vi "4 way traffic light system.vi"() -> ()   [LabVIEW 2021]
panel:
  in  "?":bool
  out "GREEN-S":bool
  out "YELLOW-S":bool
  out "RED-S":bool
  out "GREEN-N":bool
  out "YELLOW-N":bool
  out "RED-N":bool
  out "GREEN-E":bool
  out "YELLOW-E":bool
  out "RED-E":bool
  out "GREEN-W":bool
  out "YELLOW-W":bool
  out "RED-W":bool
  # "-----------------------------------------------------------------------------"
  # "----------------------------------------------------------------"
  # "----------------------------------------------------------------"
  # "------------------------------------------------------------------------"
  # "-------------------------------------------------------------"
  # "-----------------------------------------------------------------------"
  # "---------------------------------------------------------------"
  # "---------------------------------------------------------------"
  # "-------------------------------------------------------------------------"
  # "--------------------------------------------"
  # "-----------------------------------------------"
  # "---------------------------------------------------"
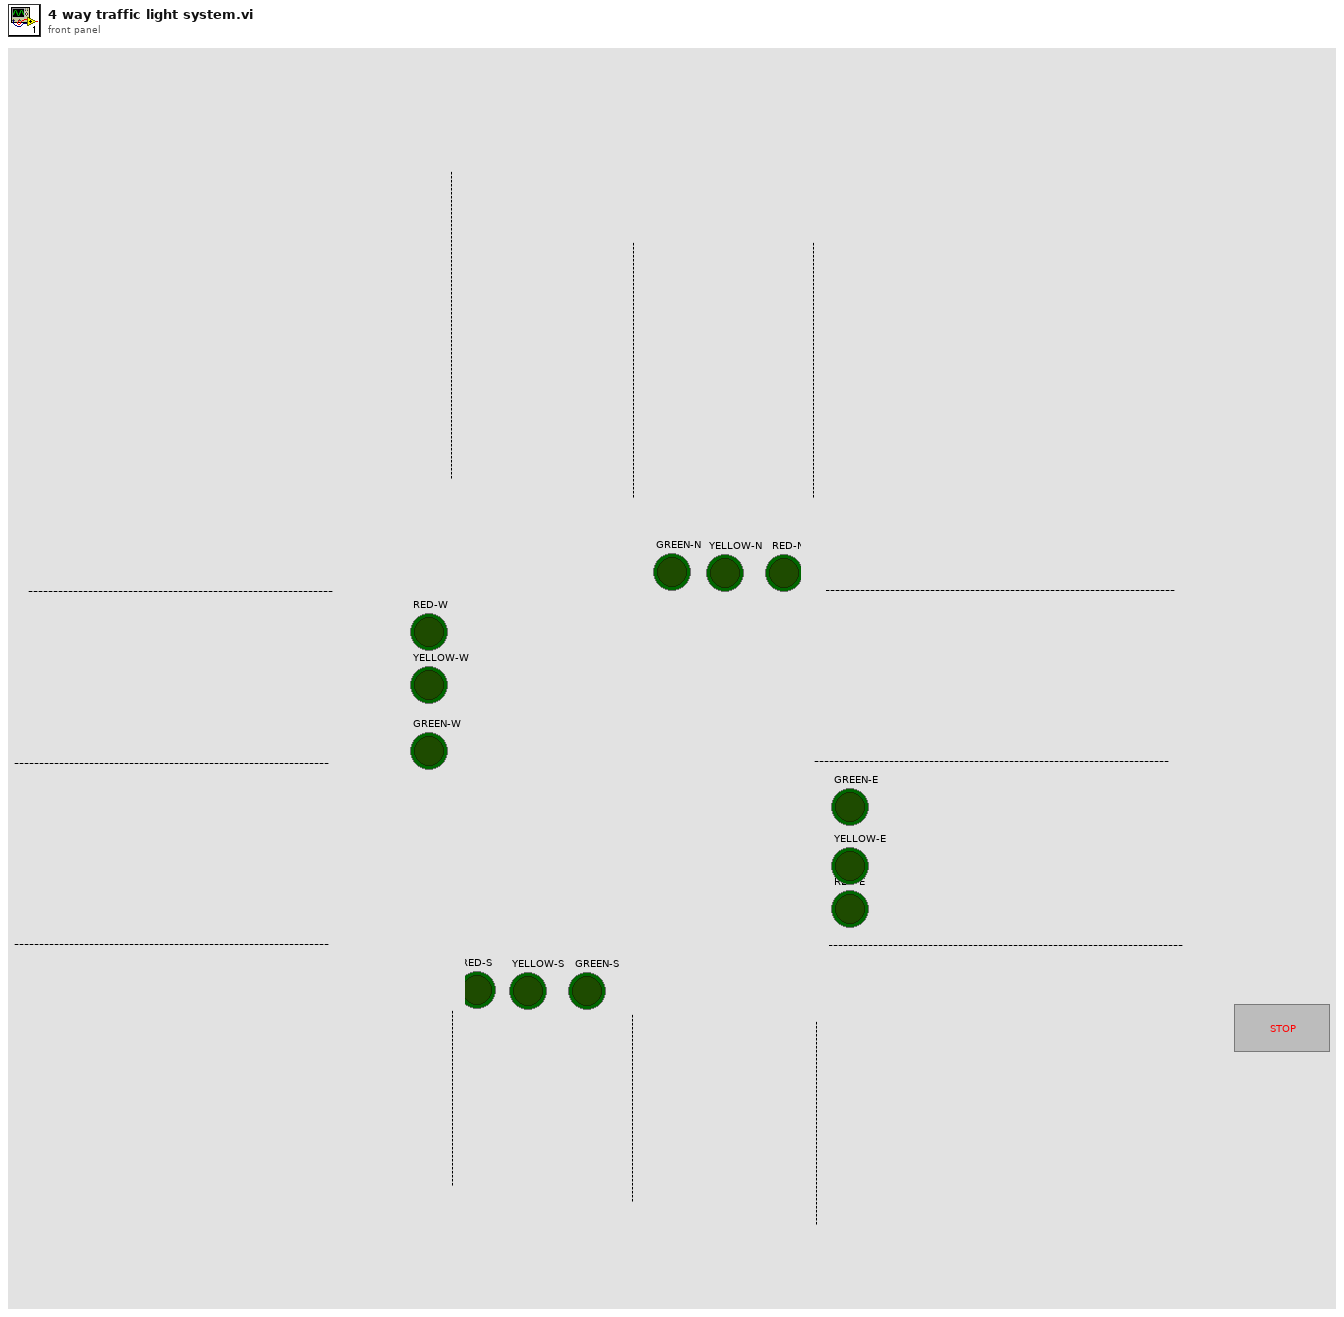
[diagram p1: front panel]
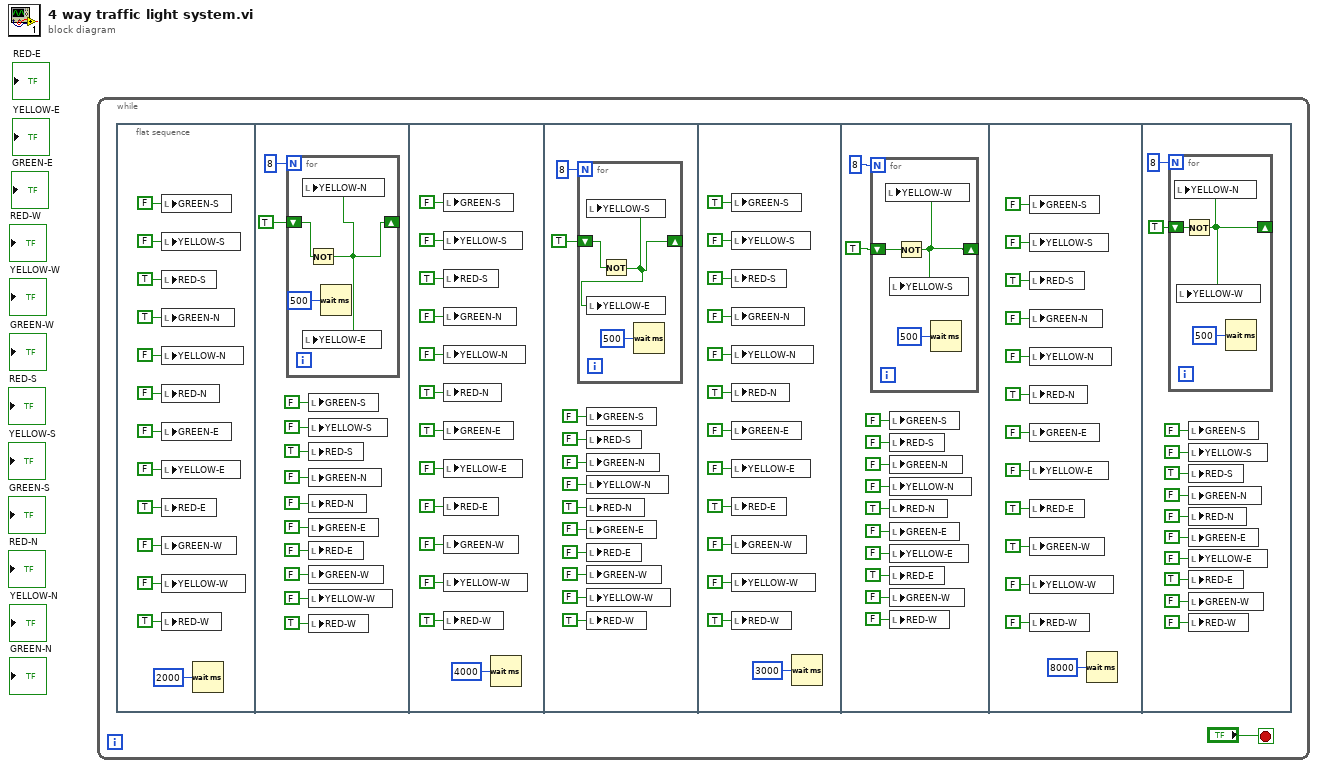
[diagram p0: block diagram]
diagram:
  n1 = while {
    stop <- "?" stop-if-true
    n2 = flat-sequence {
      frame #0 {
        n3 = local write "GREEN-S"(FALSE ("GREEN-S")) -> ()
        n4 = local write "YELLOW-S"(FALSE ("YELLOW-S")) -> ()
        n5 = local write "RED-S"(TRUE ("RED-S")) -> ()
        n6 = local write "GREEN-N"(TRUE ("GREEN-N")) -> ()
        n7 = local write "YELLOW-N"(FALSE ("YELLOW-N")) -> ()
        n8 = local write "RED-N"(FALSE ("RED-N")) -> ()
        n9 = local write "GREEN-E"(FALSE ("GREEN-E")) -> ()
        n10 = local write "YELLOW-E"(FALSE ("YELLOW-E")) -> ()
        n11 = local write "RED-E"(TRUE ("RED-E")) -> ()
        n12 = local write "GREEN-W"(FALSE ("GREEN-W")) -> ()
        n13 = local write "YELLOW-W"(FALSE ("YELLOW-W")) -> ()
        n14 = local write "RED-W"(TRUE ("RED-W")) -> ()
        n15 = Wait (ms)(milliseconds to wait=u32 2000) -> ()  [unwired: 1 out]
      }
      frame #1 {
        n16 = for {
          N: 8 -> [_]
          shift-right: [w27] -> _
          shift-left: TRUE -> [w28]
          n17 = Not(x=w28) -> (.not. x?=w27:bool)
          n18 = local write "YELLOW-N"(w27) -> ()
          n19 = local write "YELLOW-E"(w27) -> ()
          n20 = Wait (ms)(milliseconds to wait=u32 500) -> ()  [unwired: 1 out]
        }
        n21 = local write "GREEN-S"(FALSE ("GREEN-S")) -> ()
        n22 = local write "YELLOW-S"(FALSE ("YELLOW-S")) -> ()
        n23 = local write "RED-S"(TRUE ("RED-S")) -> ()
        n24 = local write "GREEN-N"(FALSE ("GREEN-N")) -> ()
        n25 = local write "RED-N"(FALSE ("RED-N")) -> ()
        n26 = local write "GREEN-E"(FALSE ("GREEN-E")) -> ()
        n27 = local write "RED-E"(FALSE ("RED-E")) -> ()
        n28 = local write "GREEN-W"(FALSE ("GREEN-W")) -> ()
        n29 = local write "YELLOW-W"(FALSE ("YELLOW-W")) -> ()
        n30 = local write "RED-W"(TRUE ("RED-W")) -> ()
      }
      frame #2 {
        n31 = local write "GREEN-S"(FALSE ("GREEN-S")) -> ()
        n32 = local write "YELLOW-S"(FALSE ("YELLOW-S")) -> ()
        n33 = local write "RED-S"(TRUE ("RED-S")) -> ()
        n34 = local write "GREEN-N"(FALSE ("GREEN-N")) -> ()
        n35 = local write "YELLOW-N"(FALSE ("YELLOW-N")) -> ()
        n36 = local write "RED-N"(TRUE ("RED-N")) -> ()
        n37 = local write "GREEN-E"(TRUE ("GREEN-E")) -> ()
        n38 = local write "YELLOW-E"(FALSE ("YELLOW-E")) -> ()
        n39 = local write "RED-E"(FALSE ("RED-E")) -> ()
        n40 = local write "GREEN-W"(FALSE ("GREEN-W")) -> ()
        n41 = local write "YELLOW-W"(FALSE ("YELLOW-W")) -> ()
        n42 = local write "RED-W"(TRUE ("RED-W")) -> ()
        n43 = Wait (ms)(milliseconds to wait=u32 4000) -> ()  [unwired: 1 out]
      }
      frame #3 {
        n44 = for {
          N: 8 -> [_]
          shift-right: [w55] -> _
          shift-left: TRUE -> [w57]
          n45 = Not(x=w57) -> (.not. x?=w55:bool)
          n46 = local write "YELLOW-S"(w55) -> ()
          n47 = local write "YELLOW-E"(w55) -> ()
          n48 = Wait (ms)(milliseconds to wait=u32 500) -> ()  [unwired: 1 out]
        }
        n49 = local write "GREEN-S"(FALSE ("GREEN-S")) -> ()
        n50 = local write "RED-S"(FALSE ("RED-S")) -> ()
        n51 = local write "GREEN-N"(FALSE ("GREEN-N")) -> ()
        n52 = local write "YELLOW-N"(FALSE ("YELLOW-N")) -> ()
        n53 = local write "RED-N"(TRUE ("RED-N")) -> ()
        n54 = local write "GREEN-E"(FALSE ("GREEN-E")) -> ()
        n55 = local write "RED-E"(FALSE ("RED-E")) -> ()
        n56 = local write "GREEN-W"(FALSE ("GREEN-W")) -> ()
        n57 = local write "YELLOW-W"(FALSE ("YELLOW-W")) -> ()
        n58 = local write "RED-W"(TRUE ("RED-W")) -> ()
      }
      frame #4 {
        n59 = local write "GREEN-S"(TRUE ("GREEN-S")) -> ()
        n60 = local write "YELLOW-S"(FALSE ("YELLOW-S")) -> ()
        n61 = local write "RED-S"(FALSE ("RED-S")) -> ()
        n62 = local write "GREEN-N"(FALSE ("GREEN-N")) -> ()
        n63 = local write "YELLOW-N"(FALSE ("YELLOW-N")) -> ()
        n64 = local write "RED-N"(TRUE ("RED-N")) -> ()
        n65 = local write "GREEN-E"(FALSE ("GREEN-E")) -> ()
        n66 = local write "YELLOW-E"(FALSE ("YELLOW-E")) -> ()
        n67 = local write "RED-E"(TRUE ("RED-E")) -> ()
        n68 = local write "GREEN-W"(FALSE ("GREEN-W")) -> ()
        n69 = local write "YELLOW-W"(FALSE ("YELLOW-W")) -> ()
        n70 = local write "RED-W"(TRUE ("RED-W")) -> ()
        n71 = Wait (ms)(milliseconds to wait=u32 3000) -> ()  [unwired: 1 out]
      }
      frame #5 {
        n72 = for {
          N: 8 -> [_]
          shift-right: [w83] -> _
          shift-left: TRUE -> [w85]
          n73 = Not(x=w85) -> (.not. x?=w83:bool)
          n74 = local write "YELLOW-W"(w83) -> ()
          n75 = local write "YELLOW-S"(w83) -> ()
          n76 = Wait (ms)(milliseconds to wait=u32 500) -> ()  [unwired: 1 out]
        }
        n77 = local write "GREEN-S"(FALSE ("GREEN-S")) -> ()
        n78 = local write "RED-S"(FALSE ("RED-S")) -> ()
        n79 = local write "GREEN-N"(FALSE ("GREEN-N")) -> ()
        n80 = local write "YELLOW-N"(FALSE ("YELLOW-N")) -> ()
        n81 = local write "RED-N"(TRUE ("RED-N")) -> ()
        n82 = local write "GREEN-E"(FALSE ("GREEN-E")) -> ()
        n83 = local write "YELLOW-E"(FALSE ("YELLOW-E")) -> ()
        n84 = local write "RED-E"(TRUE ("RED-E")) -> ()
        n85 = local write "GREEN-W"(FALSE ("GREEN-W")) -> ()
        n86 = local write "RED-W"(FALSE ("RED-W")) -> ()
      }
      frame #6 {
        n87 = local write "GREEN-S"(FALSE ("GREEN-S")) -> ()
        n88 = local write "YELLOW-S"(FALSE ("YELLOW-S")) -> ()
        n89 = local write "RED-S"(TRUE ("RED-S")) -> ()
        n90 = local write "GREEN-N"(FALSE ("GREEN-N")) -> ()
        n91 = local write "YELLOW-N"(FALSE ("YELLOW-N")) -> ()
        n92 = local write "RED-N"(TRUE ("RED-N")) -> ()
        n93 = local write "GREEN-E"(FALSE ("GREEN-E")) -> ()
        n94 = local write "YELLOW-E"(FALSE ("YELLOW-E")) -> ()
        n95 = local write "RED-E"(TRUE ("RED-E")) -> ()
        n96 = local write "GREEN-W"(TRUE ("GREEN-W")) -> ()
        n97 = local write "YELLOW-W"(FALSE ("YELLOW-W")) -> ()
        n98 = local write "RED-W"(FALSE ("RED-W")) -> ()
        n99 = Wait (ms)(milliseconds to wait=u32 8000) -> ()  [unwired: 1 out]
      }
      frame #7 {
        n100 = for {
          N: 8 -> [_]
          shift-right: [w111] -> _
          shift-left: TRUE -> [w113]
          n101 = Not(x=w113) -> (.not. x?=w111:bool)
          n102 = local write "YELLOW-N"(w111) -> ()
          n103 = local write "YELLOW-W"(w111) -> ()
          n104 = Wait (ms)(milliseconds to wait=u32 500) -> ()  [unwired: 1 out]
        }
        n105 = local write "GREEN-S"(FALSE ("GREEN-S")) -> ()
        n106 = local write "YELLOW-S"(FALSE ("YELLOW-S")) -> ()
        n107 = local write "RED-S"(TRUE ("RED-S")) -> ()
        n108 = local write "GREEN-N"(FALSE ("GREEN-N")) -> ()
        n109 = local write "RED-N"(FALSE ("RED-N")) -> ()
        n110 = local write "GREEN-E"(FALSE ("GREEN-E")) -> ()
        n111 = local write "YELLOW-E"(FALSE ("YELLOW-E")) -> ()
        n112 = local write "RED-E"(TRUE ("RED-E")) -> ()
        n113 = local write "GREEN-W"(FALSE ("GREEN-W")) -> ()
        n114 = local write "RED-W"(FALSE ("RED-W")) -> ()
      }
    }
  }
